vi "Cylindrical to Cartesian.vi"(4 "Cylindrical\nCoordinates":cluster{"r":dbl, "theta":dbl, "z":dbl}) -> (1 "Cartesian\nCoordinates":cluster{"x":dbl, "y":dbl, "z":dbl})   [LabVIEW 2013]
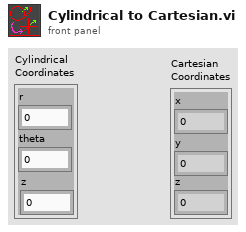
[diagram p1: front panel]
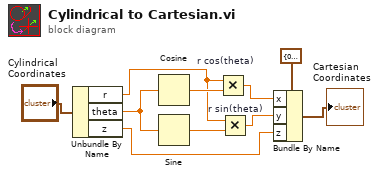
[diagram p0: block diagram]
diagram:
  n1 = Unbundle By Name("Cylindrical\nCoordinates") -> ("r"=w2:dbl, "theta"=w3:dbl, "z"=w1:dbl)
  n2 = Cosine(x=w3) -> (cos(x)=w10:dbl)
  n3 = Sine(x=w3) -> (sin(x)=w9:dbl)
  n4 = Multiply "r cos(theta)"(x=w2, y=w10) -> (x*y=w6:dbl)
  n5 = Multiply "r sin(theta)"(x=w2, y=w9) -> (x*y=w5:dbl)
  n6 = Bundle By Name(cluster=cluster{"x":dbl, "y":dbl, "z":dbl} {"x"=0.0, "y"=0.0, "z"=0.0} ("input cluster"), "x"=w6, "y"=w5, "z"=w1) -> (→"Cartesian\nCoordinates":cluster{"x":dbl, "y":dbl, "z":dbl})
